vi "ElevatorBrake.vi"(1 "Power In":dbl) -> (0 "Power Out":dbl)   [LabVIEW 2018]
uses:
  <vilib>/Rock Robotics/WPI/Solenoid/WPI_SolenoidValue.ctl
  <vilib>/Rock Robotics/WPI/Solenoid/WPI_SolenoidSetEnum.vi
panel:
  in  "Outter Upper limit":dbl=0.1 format="%#_13g"
  in  "Outter Lower limit":dbl=-0.3 format="%#_13g"
  in  "Inner Upper limit":dbl=0.1 format="%#_13g"
  in  "Inner Lower limit":dbl=-0.25 format="%#_13g"
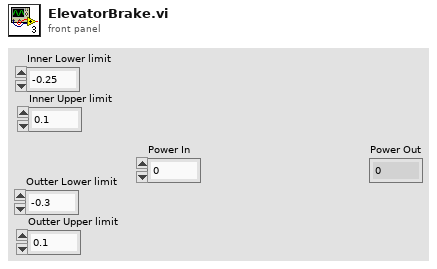
[diagram p1: front panel]
types:
  T1 = typedef "WPI_SolenoidValue.ctl" = enum16{"Off", "On", "Forward", "Reverse"}
  T2 = typedef "WPI_SolenoidDevRef.ctl" = cluster{"DevStatus":errorcluster, "Pneumatics Control Module":u8, "Forward Solenoid Channel":T3, "Reverse Solenoid Channel":T3}
  T3 = typedef "WPI_SolenoidChannel.ctl" = enum8{"Solenoid 0", "Solenoid 1", "Solenoid 2", "Solenoid 3", "Solenoid 4", "Solenoid 5", "Solenoid 6", "Solenoid 7", "Invalid"}
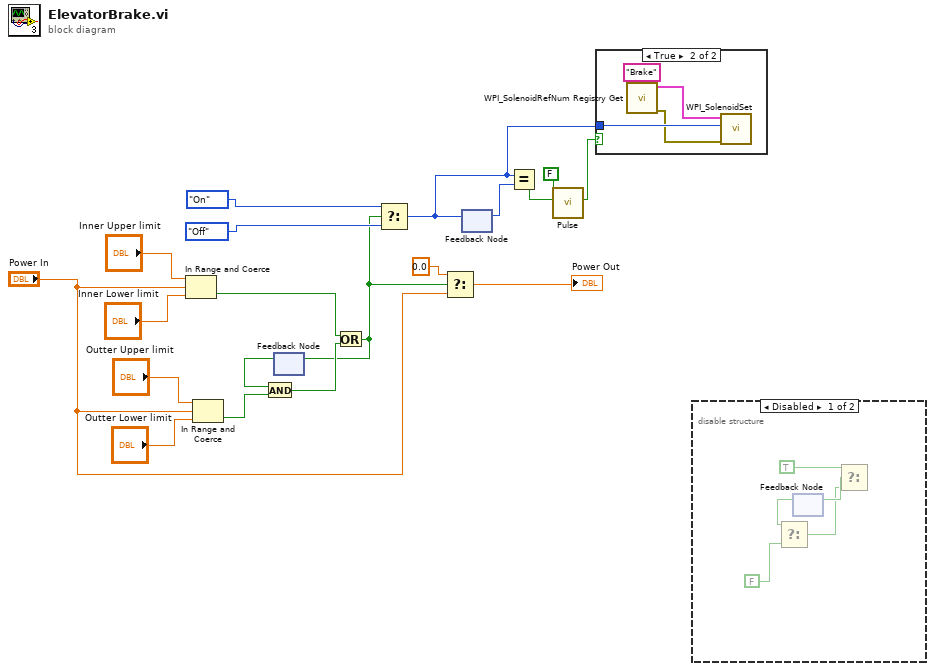
[diagram p0: block diagram]
diagram:
  n1 = In Range and Coerce(upper limit="Inner Upper limit", x="Power In", lower limit="Inner Lower limit") -> (In Range?=w2:bool)  [unwired: 1 out]
  n2 = In Range and Coerce(upper limit="Outter Upper limit", x="Power In", lower limit="Outter Lower limit") -> (In Range?=w3:bool)  [unwired: 1 out]
  n3 = feedback #1() -> (w4:bool)  [unwired: 1 in]
  n4 = And(x=w4, y=w3) -> (x .and. y?=w5:bool)
  n5 = Or(x=w2, y=w5) -> (x .or. y?=w1:bool)
  n6 = feedback-in #1(w1) -> ()
  n7 = Select(t=WPI_SolenoidValue."On" ("Value"), s=w1, f=WPI_SolenoidValue."Off" ("Value")) -> (s? t:f=w9:T1)
  n8 = Select(t=0.0, s=w1, f="Power In") -> (s? t:f=→"Power Out":dbl)
  n9 = feedback-in #2(w9) -> ()
  n10 = feedback #2() -> (w10:T1)  [unwired: 1 in]
  n11 = Equal?(x=w9, y=w10) -> (x = y?=w11:bool)
  n12 = call "Pulse.vi"("Input"=w11, "Rising Edge?"=FALSE) -> ("Output"=w15:bool)  [unwired: 9 in]
  n13 = case shown="True" w15 {
    tunnel: w9 -> [_ w23]
    frame False {
    }
    frame True {
      n14 = call <vilib>:"WPI_SolenoidRefNum Registry Get.vi"("refnum name"="Brake") -> ("error out"=w20:errorcluster, "SolenoidDevRef"=w21:T2)  [unwired: 9 in]
      n15 = call-poly <vilib>:"WPI_SolenoidSet.vi"("error in (no error)"=w20, "Value"=w23, "SolenoidDevRef"=w21) -> ()  [unwired: 7 in, 2 out]
    }
  }
  n16 = disable-structure shown="Disabled" {
    frame Disabled {
      n17 = feedback #3() -> (w29:bool)  [unwired: 1 in]
      n18 = Select(t=w29, f=FALSE) -> (s=w26:bool, s? t:f=w24:bool)
      n19 = Select(t=TRUE, f=w24) -> (s=w25:bool, s? t:f=w30:bool)
      n20 = feedback-in #3(w30) -> ()
    }
    frame Enabled {
    }
  }
